vi "Timing.vi"() -> ()   [LabVIEW 2020]
uses:
  <vilib>/Platform/TimedLoop/XDataNode/timing_clust.ctl
  <vilib>/Platform/TimedLoop/XDataNode/nitl_modes.ctl
  <vilib>/Platform/TimedLoop/XDataNode/wakeup.ctl
  <vilib>/Platform/TimedLoop/XDataNode/XDataNode.xnode
  <vilib>/Platform/TimedLoop/XDataNode/XDNodeRunTimeDep.lvlib
panel:
  out "Graph":i32[][](graph)
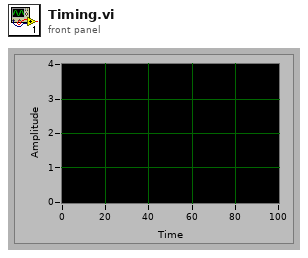
[diagram p1: front panel]
types:
  T1 = typedef "XDNodeRunTimeDep.lvlib/timing_clust.ctl" = cluster{"Expected End [f-1]":u64, "Actual End [f-1]":u64, "Finished Late? [f-1]":bool, "Expected End [i-1]":u64, "Actual End [i-1]":u64, "Finished Late? [i-1]":bool, "Expected Start [i]":u64, "Actual Start [i]":u64, "Expected Start [f]":u64, "Actual Start [f]":u64, "Source Name":string, "Structure Name":string, "Period":i64, "Deadline":i64, "Offset":i64, "Start":i64, "Priority":i32, "Timeout":i32, "Mode":T2, "Wakeup Reason":T3, "Error":errorcluster, "Source Type":string, "Secondary Source Type":string, "Global End Time":u64, "Global Start Time":u64, "Frame Duration":u64, "Iteration Duration":u64, "Assigned CPU":i32, "I/O Scan Engine Mode":u32}
  T2 = typedef "XDNodeRunTimeDep.lvlib/nitl_modes.ctl" = enum32{"No Change", "Process missed periods, maintain original phase", "Discard missed periods, maintain original phase", "Process missed periods, ignore original phase", "Discard missed periods, ignore original phase"}
  T3 = typedef "XDNodeRunTimeDep.lvlib/wakeup.ctl" = enum32{"Normal", "Aborted", "Asynchronous wakeup", "Timing source error", "Timed loop error", "Timeout"}
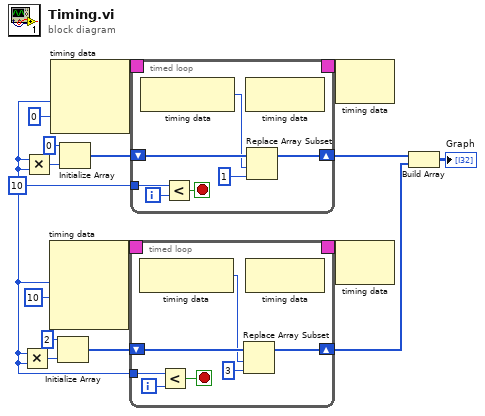
[diagram p0: block diagram]
diagram:
  w3 = 10
  n1 = Multiply(x=w3, y=w3) -> (x*y=w8:i32)
  n2 = Multiply(x=w3, y=w3) -> (x*y=w11:i32)
  n3 = node-c288(w3, i64 10 ("Offset")) -> (w14:T1)  [unwired: 2 in]
  n4 = node-c288(w3, i64 0 ("Offset")) -> (w16:T1)  [unwired: 1 in]
  n5 = Initialize Array(2, w8) -> (w7:i32[])
  n6 = Initialize Array(0, w11) -> (w5:i32[])
  n7 = timed-loop {
    timing: w14 -> [_]
    timing-out: [_] -> w13
    tunnel: w3 -> [w22]
    shift-right: [w18] -> w4
    shift-left: w7 -> [w19]
    i -> [w23]
    stop <- w21 stop-if-true
    n8 = node-c288() -> (w17:i64)  [unwired: 1 in]
    n9 = Less?(x=w22, y=w23) -> (x < y?=w21:bool)
    n10 = Replace Array Subset(array=w19, new element=3 ("new element/subarray"), index=w17) -> (w18:i32[])
    n11 = node-c288() -> ()  [unwired: 1 in, 1 out]
  }
  n12 = timed-loop {
    timing: w16 -> [_]
    timing-out: [_] -> w15
    tunnel: w3 -> [w33]
    shift-right: [w29] -> w6
    shift-left: w5 -> [w30]
    i -> [w32]
    stop <- w31 stop-if-true
    n13 = node-c288() -> (w28:i64)  [unwired: 1 in]
    n14 = Less?(x=w33, y=w32) -> (x < y?=w31:bool)
    n15 = node-c288() -> ()  [unwired: 1 in, 1 out]
    n16 = Replace Array Subset(array=w30, new element=1 ("new element/subarray"), index=w28) -> (w29:i32[])
  }
  n17 = node-c288(w15) -> ()  [unwired: 1 out]
  n18 = node-c288(w13) -> ()  [unwired: 1 out]
  n19 = Build Array(w6, w4) -> (→"Graph":i32[][])
